vi "End.vi"(8 "error in (no error)":errorcluster, 11 "Experiment2D in":refnum<class "Experiment2D.lvclass">) -> (0 "error out":errorcluster, 3 "Experiment2D out":refnum<class "Experiment2D.lvclass">)   [LabVIEW 2018, in "Experiment2D.lvclass"]
uses:
  Experiment2D.lvclass
  Experiment2D.lvclass/Experiment2D.ctl
  Measurement/Measurement2D/Measurement2D.lvclass
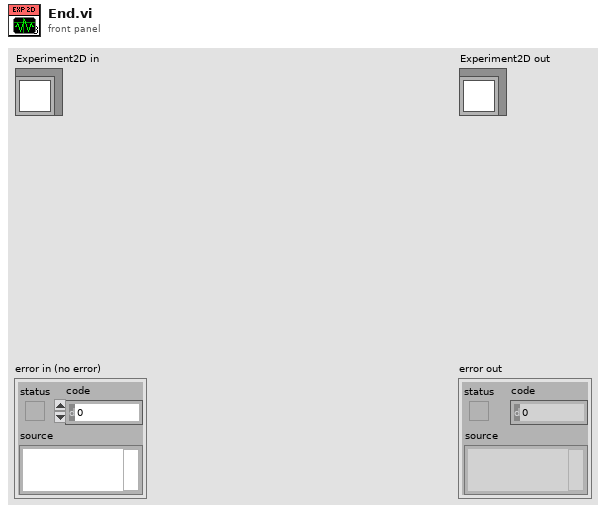
[diagram p1: front panel]
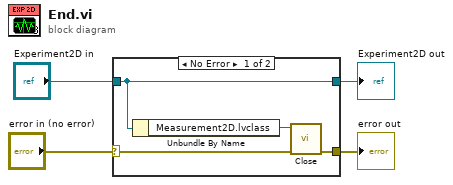
[diagram p0: block diagram]
diagram:
  n1 = case shown="No Error" "error in (no error)" {
    selector: "error in (no error)" -> [w6 w10]
    tunnel: [w5 w10] -> w3
    tunnel: [w8 w9] -> w1
    tunnel: "Experiment2D in" -> [w8 w9]
    frame No Error {
      n2 = Unbundle By Name(w8) -> ("Measurement2D.lvclass"=w7:refnum<class "Measurement2D.lvclass">)
      n3 = call-dynamic "Close.vi"("error in (no error)"=w6, "Measurement2D in"=w7) -> ("error out"=w5:errorcluster)  [unwired: 8 in, 1 out]
    }
    frame Error {
    }
  }
  "error out" <- w3
  "Experiment2D out" <- w1
